vi "Tank Drive.vi"(0 "LeftActual":dbl, 1 "MotorName":string="TankDrive", 2 "DriveAction":T1, 5 "Right Actual":dbl, 7 "LeftDesired":dbl, 9 "RightDesired":dbl, 11 "error in (no error)":errorcluster, 12 "LoopTime":dbl, 13 "AccelRate":dbl) -> (4 "LeftOut":dbl, 6 "RightOut":dbl, 15 "error out":errorcluster)   [LabVIEW 2013]
doc: "Straight drive True locks both motor desired values to the left joystick.\nHalf drive True divides desired values by 2 to allow more fine controls. This does not half the accel rate."
uses:
  DriveAction.ctl
  <vilib>/Rock Robotics/WPI/RobotDrive/WPI_RobotDriveGetSetRefNum.vi
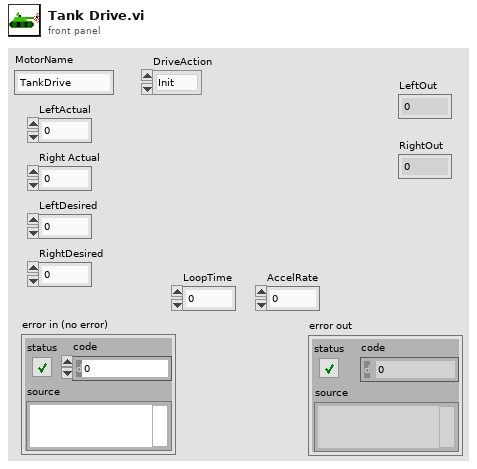
[diagram p1: front panel]
types:
  T1 = typedef "DriveAction.ctl" = enum16{"Init", "LinearDrive", "SetValue", "Disable"}
  T2 = typedef "WPI_RobotDriveDevRef.ctl" = cluster{"DevStatus":errorcluster, "Motors[]":T3[], "Square Inputs":bool, "Max Output":dbl, "Isochronous":bool}
  T3 = typedef "WPI_MotorControlDeviceRef.ctl" = cluster{"DeviceStatus":errorcluster, "Type":enum16{"PWM", "CAN"}, "PWM":cluster{"Digital Module":T4, "PWM Channel":T5, "DeadBand":T6}, "CAN":cluster{"Device Number":u8, "Control Mode":T7, "Semaphore":T8, "Max Vout":dbl}, "Invert":bool, "TransformRef":T9, "InvTransformRef":T9}
  T4 = typedef "FPGA_TypedefDigitalModule.ctl" = enum16{"Digital Module 1", "Digital Module 2"}
  T5 = typedef "FPGA_DIOPWMChannel.ctl" = enum8{"PWM 1", "PWM 2", "PWM 3", "PWM 4", "PWM 5", "PWM 6", "PWM 7", "PWM 8", "PWM 9", "PWM 10", "Invalid"}
  T6 = typedef "WPI_PWMDeadband.ctl" = cluster{"Name":string, "maxPositivePwm":i32, "minPositivePwm":i32, "centerPwm":i32, "maxNegativePwm":i32, "minNegativePwm":i32, "angularRange":u16}
  T7 = typedef "WPI_CANJaguar_ControlMode.ctl" = enum8{"Percent VBus", "Current", "Speed", "Position", "Voltage"}
  T8 = typedef "Semaphore RefNum" = refnum<k1>
  T9 = typedef "WPI_PWMTransform_ConPane.ctl" = refnum<vi>
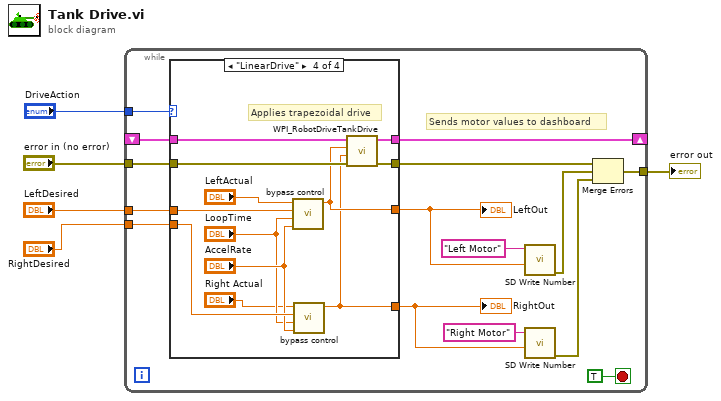
[diagram p0: block diagram]
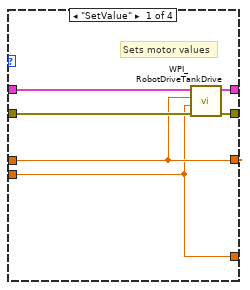
[diagram p2: hidden frame]
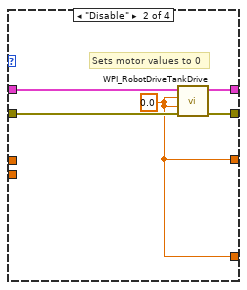
[diagram p3: hidden frame]
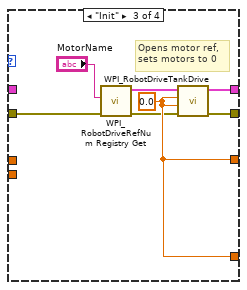
[diagram p4: hidden frame]
diagram:
  n1 = while {
    shift-right: [w20] -> _
    shift-left: _ -> [w18]
    tunnel: [w15] -> w5
    tunnel: "error in (no error)" -> [w12]
    tunnel: "DriveAction" -> [w10]
    tunnel: "LeftDesired" -> [w7]
    tunnel: "RightDesired" -> [w6]
    stop <- TRUE stop-if-true
    # "Sends motor values to dashboard"
    n2 = case shown="\"LinearDrive\"" w10 {
      tunnel: [w21 w30 w33 w40] -> w20
      tunnel: w18 -> [w22 w31 _ w39]
      tunnel: w12 -> [w26 w29 w38 w49]
      tunnel: [w25 w28 w37 w50] -> w11
      tunnel: [w24 w27 w36 w46] -> w9
      tunnel: [w23 w27 w36 w45] -> w8
      tunnel: w7 -> [w24 _ _ w48]
      tunnel: w6 -> [w23 _ _ w47]
      frame "SetValue" {
        # "Sets motor values"
        n3 = call <vilib>:"WPI_RobotDriveTankDrive.vi"("error in (no error)"=w26, "Right axis value"=w23, "Left axis value"=w24, "RobotDriveDevRef"=w22) -> ("error out"=w25:errorcluster, "RobotDriveDevRef"=w21:T2)  [unwired: 5 in, 1 out]
      }
      frame "Disable" {
        w27 = 0.0
        # "Sets motor values to 0"
        n4 = call <vilib>:"WPI_RobotDriveTankDrive.vi"("error in (no error)"=w29, "Right axis value"=w27, "Left axis value"=w27, "RobotDriveDevRef"=w31) -> ("error out"=w28:errorcluster, "RobotDriveDevRef"=w30:T2)  [unwired: 5 in, 1 out]
      }
      frame "Init" {
        w36 = 0.0
        # "Opens motor ref,\nsets motors to 0"
        n5 = call <vilib>:"WPI_RobotDriveRefNum Registry Get.vi"("error in (no error)"=w38, "refnum name"="MotorName") -> ("error out"=w34:errorcluster, "RobotDriveDevRef"=w35:T2)  [unwired: 8 in]
        n6 = call <vilib>:"WPI_RobotDriveTankDrive.vi"("error in (no error)"=w34, "Right axis value"=w36, "Left axis value"=w36, "RobotDriveDevRef"=w35) -> ("error out"=w37:errorcluster, "RobotDriveDevRef"=w33:T2)  [unwired: 5 in, 1 out]
      }
      frame "LinearDrive" {
        # "Applies trapezoidal drive"
        n7 = call "bypass control.vi"("AccelRate"="AccelRate", "LoopTime"="LoopTime", "Joystick"=w48, "MotorInput"="LeftActual") -> ("SetMotor"=w46:dbl)  [unwired: 7 in]
        n8 = call "bypass control.vi"("AccelRate"="AccelRate", "LoopTime"="LoopTime", "Joystick"=w47, "MotorInput"="Right Actual") -> ("SetMotor"=w45:dbl)  [unwired: 7 in]
        n9 = call <vilib>:"WPI_RobotDriveTankDrive.vi"("error in (no error)"=w49, "Right axis value"=w45, "Left axis value"=w46, "RobotDriveDevRef"=w39) -> ("error out"=w50:errorcluster, "RobotDriveDevRef"=w40:T2)  [unwired: 5 in, 1 out]
      }
    }
    "RightOut" <- w8
    "LeftOut" <- w9
    n10 = call <vilib>:"SD Write Number.vi"("Numeric"=w9, "Name"="Left Motor") -> ("error out"=w14:errorcluster)  [unwired: 8 in, 1 out]
    n11 = call <vilib>:"SD Write Number.vi"("Numeric"=w8, "Name"="Right Motor") -> ("error out"=w13:errorcluster)  [unwired: 8 in, 1 out]
    n12 = Merge Errors(w11, w14, w13) -> (w15:errorcluster)
  }
  "error out" <- w5
